vi "AQICalc.vi"(7 "ChosenRange":i32, 8 "error in (no error)":errorcluster, 9 "PMMeasurement":dbl, 10 "BP high PM":dbl[](array[numeric])=[12.0, 35.4, 55.4, 150.4, 250.4, 350.4, 500.4], 11 "BP low PM":dbl[](array[numeric])=[0.0, 12.1, 35.5, 55.5, 150.5, 250.5, 350.5]) -> (0 "error out":errorcluster, 3 "AQI":dbl)   [LabVIEW 2013]
doc: "Use this template to build a VI to use as a subVI."
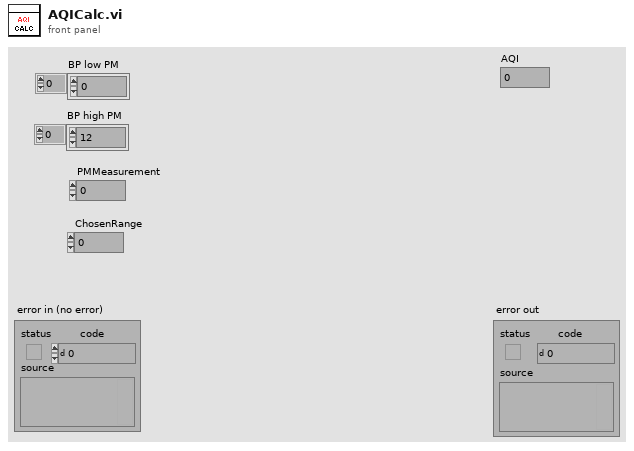
[diagram p1: front panel]
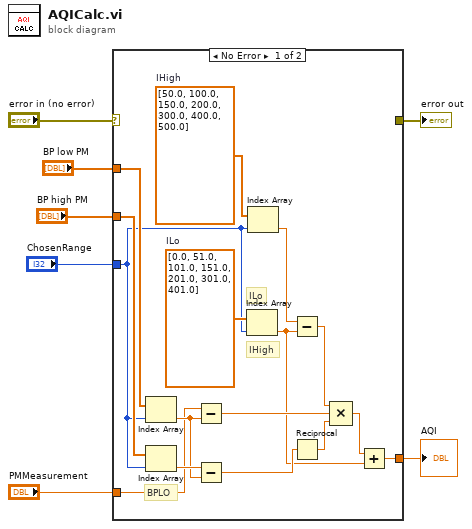
[diagram p0: block diagram]
diagram:
  n1 = case shown="No Error" "error in (no error)" {
    selector: "error in (no error)" -> [_ w24]
    tunnel: [_ w24] -> w6
    tunnel: "BP low PM" -> [w12 _]
    tunnel: "BP high PM" -> [w11 _]
    tunnel: "PMMeasurement" -> [w10 _]
    tunnel: "ChosenRange" -> [w9 _]
    tunnel: [w8 _] -> w1
    frame No Error {
      w14 = dbl[] [50.0, 100.0, 150.0, 200.0, 300.0, 400.0, 500.0]  # IHigh
      w13 = dbl[] [0.0, 51.0, 101.0, 151.0, 201.0, 301.0, 401.0]  # ILo
      # "BPLO"
      # "IHigh"
      # "ILo"
      n2 = Index Array(array=w12, index=w9) -> (element=w21:dbl)
      n3 = Index Array(array=w11, index=w9) -> (element=w22:dbl)
      n4 = Subtract(x=w10, y=w21) -> (x-y=w18:dbl)
      n5 = Subtract(x=w22, y=w21) -> (x-y=w20:dbl)
      n6 = Index Array(array=w13, index=w9) -> (element=w15:dbl)
      n7 = Index Array(array=w14, index=w9) -> (element=w23:dbl)
      n8 = Subtract(x=w23, y=w15) -> (x-y=w17:dbl)
      n9 = Reciprocal(x=w20) -> (1/x=w19:dbl)
      n10 = Compound Arithmetic op=MULTIPLY(w17, w18, w19) -> (w16:dbl)
      n11 = Add(x=w16, y=w15) -> (x+y=w8:dbl)
    }
    frame Error {
    }
  }
  "error out" <- w6
  "AQI" <- w1
